vi "Lancing 2 Integ.vi"(0 "Image Out":T8(plugin-control), 1 "REF ROI":T4 {"Contours"."Type" items=["No Selection", "Point", "Line", "Rectangle", "Oval", "Polygon", "Free", "Annulus", "Unused2", "Unused3", "Broken Line", "Free Hand Line", "Rotated Rectangle"]}, 2 "Edge Options Ref ROI":T2={"Edge Polarity"=2, "Kernel Size"=5, "Width"=5, "Minimum Edge Strength"=50.0, "Interpolation Type"=enum."Bilinear Fixed", "Data Processing Method"=enum."Average"} {"Edge Polarity" items=["All Edges", "Rising Edges", "Falling Edges"]; "Minimum Edge Strength" format="%.2f"; "Width" step=2; "Kernel Size" step=2}, 3 "Search Direction Ref ROI":u32(ring)=2 items=["Left to Right", "Right to Left", "Top to Bottom", "Bottom to Top"], 4 "Line Options Ref ROI":T6={"Number of Lines"=1, "Type"=enum."First Edge Rake", "Min. Score"=10.0, "Max. Score"=1000.0, "Orientation"=0.0, "Angle Range"=30.0, "Angle Tolerance"=5.0, "Step Size"=3, "Min. SNR (db)"=0.0, "Min. Points (%)"=25.0, "Hough Iterations"=5} {"Min. Points (%)" min=0.0 max=100.0; "Min. SNR (db)" min=0.0; "Max. Score" min=0.0 max=1024.0; "Min. Score" min=0.0 max=1024.0 step=1.0}, 5 "Meas ROI 1":T4 {"Contours"."Type" items=["No Selection", "Point", "Line", "Rectangle", "Oval", "Polygon", "Free", "Annulus", "Unused2", "Unused3", "Broken Line", "Free Hand Line", "Rotated Rectangle"]}, 6 "Meas ROI 2":T4 {"Contours"."Type" items=["No Selection", "Point", "Line", "Rectangle", "Oval", "Polygon", "Free", "Annulus", "Unused2", "Unused3", "Broken Line", "Free Hand Line", "Rotated Rectangle"]}, 7 "error in (no error)":errorcluster, 8 "Calibrated Image":T8, 9 "Edge Options ROI 1":T2={"Edge Polarity"=2, "Kernel Size"=5, "Width"=5, "Minimum Edge Strength"=100.0, "Interpolation Type"=enum."Bilinear Fixed", "Data Processing Method"=enum."Average"} {"Edge Polarity" items=["All Edges", "Rising Edges", "Falling Edges"]; "Minimum Edge Strength" format="%.2f"; "Width" step=2; "Kernel Size" step=2}, 10 "Step Size ROI 1":u32=5, 11 "Process ROI 1":T1(ring), 12 "Scan Direction ROI 1":u16(ring)=3 items=["Left To Right", "Right To Left", "Top To Bottom", "Bottom To Top"], 13 "Process ROI 2":T1(ring), 14 "Step Size ROI 2":u32=1, 15 "OverlayOptions":T5, 16 "Edge Options ROI 2":T2={"Edge Polarity"=2, "Kernel Size"=9, "Width"=9, "Minimum Edge Strength"=50.0, "Interpolation Type"=enum."Bilinear Fixed", "Data Processing Method"=enum."Average"} {"Edge Polarity" items=["All Edges", "Rising Edges", "Falling Edges"]; "Minimum Edge Strength" format="%.2f"; "Width" step=2; "Kernel Size" step=2}, 17 "Scan Direction ROI 2":u16(ring)=3 items=["Left To Right", "Right To Left", "Top To Bottom", "Bottom To Top"]) -> (20 "Lancing 2":sgl, 27 "error out":errorcluster)   [LabVIEW 2019, in "Algorithm.lvclass"]
uses:
  FrameworkOverrides/Algorithm.lvclass
  <vilib>/vision/NI_Vision_Development_Module.lvlib
  <vilib>/vision/Image Controls.llb/IMAQ Image.ctl
  <vilib>/vision/Measure.llb/Edge Polarity.ctl
  <vilib>/vision/Measure.llb/Edge Options.ctl
  <vilib>/vision/Measure.llb/Straight Edge Process.ctl
  <vilib>/vision/Measure.llb/Straight Edge Options.ctl
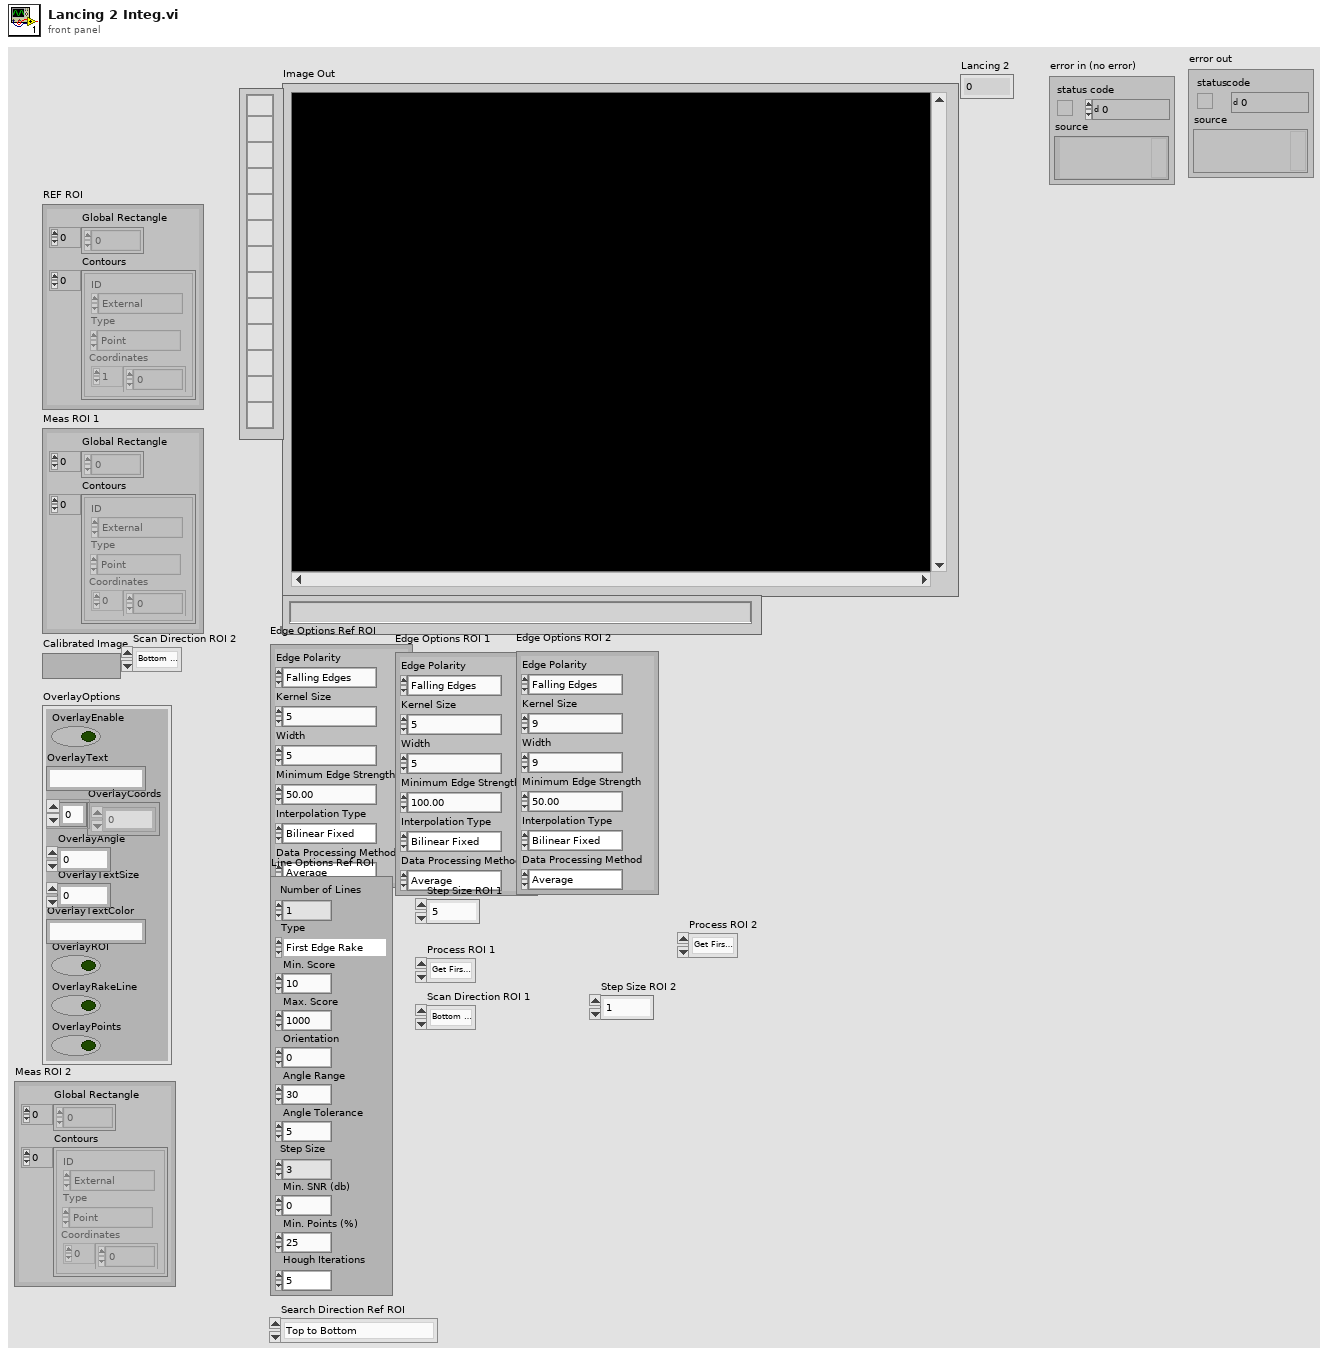
[diagram p1: front panel]
types:
  T1 = enum16{"Get First Edge", "Get First + Last Edge", "Get All Edges", "Get Best Edge"}
  T2 = typedef "Edge Options.ctl" = cluster{"Edge Polarity":T3, "Kernel Size":u32, "Width":u32, "Minimum Edge Strength":sgl, "Interpolation Type":enum32{"Zero Order", "Bilinear", "Quadratic", "Cubic", "Bilinear Fixed"}, "Data Processing Method":enum32{"Average", "Median"}}
  T3 = typedef "Edge Polarity.ctl" = u32
  T4 = cluster{"Global Rectangle":i32[], "Contours":cluster{"ID":enum32{"External", "Internal"}, "Type":u32, "Coordinates":i32[]}[]}
  T5 = cluster{"OverlayEnable":bool, "OverlayText":string, "OverlayCoords":i32[], "OverlayAngle":i32, "OverlayTextSize":i32, "OverlayTextColor":string, "OverlayROI":bool, "OverlayRakeLine":bool, "OverlayPoints":bool}
  T6 = typedef "Straight Edge Options.ctl" = cluster{"Number of Lines":i32, "Type":T7, "Min. Score":dbl, "Max. Score":dbl, "Orientation":dbl, "Angle Range":dbl, "Angle Tolerance":dbl, "Step Size":u32, "Min. SNR (db)":dbl, "Min. Points (%)":dbl, "Hough Iterations":i32}
  T7 = typedef "Straight Edge Process.ctl" = enum32{"First Edge Rake", "Best Edge Rake", "Hough Edge Rake", "First Edge Projection", "Best Edge Projection"}
  T8 = typedef "IMAQ Image.ctl" = refnum<image>
  T9 = cluster{"Point 1":cluster{"X":sgl, "Y":sgl}, "Point 2":cluster{"X":sgl, "Y":sgl}}
  T10 = typedef "IMAQ Rectangle" = cluster{"Left":i32, "Top":i32, "Right":i32, "Bottom":i32, "Rotation":dbl}
  T11 = cluster{"Point1 (Pixels)":cluster{"X":sgl, "Y":sgl}, "Point2 (Pixels)":cluster{"X":sgl, "Y":sgl}, "Point1 (Real-World)":cluster{"X":sgl, "Y":sgl}, "Point2 (Real-World)":cluster{"X":sgl, "Y":sgl}, "Angle (Pixel)":dbl, "Angle (Real-World)":dbl, "Score":dbl, "Straightness":dbl, "Average SNR (db)":dbl, "Calibration Valid":bool}[]
  T12 = typedef "Search Line.ctl" = cluster{"Start Point":cluster{"X":sgl, "Y":sgl}, "End Point":cluster{"X":sgl, "Y":sgl}, "Edge Info":T13[], "Edge Map":dbl[], "Calibration Valid":bool}
  T13 = typedef "Edge New.ctl" = cluster{"Location (Pixel)":cluster{"X":sgl, "Y":sgl}, "Location (Real-World)":cluster{"X":sgl, "Y":sgl}, "Distance (Pixel)":dbl, "Distance (Real-World)":dbl, "Strength":dbl, "Noise":dbl, "Rising?":bool}
  T14 = cluster{"Point1 (Pixels)":cluster{"X":sgl, "Y":sgl}, "Point2 (Pixels)":cluster{"X":sgl, "Y":sgl}, "Point1 (Real-World)":cluster{"X":sgl, "Y":sgl}, "Point2 (Real-World)":cluster{"X":sgl, "Y":sgl}, "Angle (Pixel)":dbl, "Angle (Real-World)":dbl, "Score":dbl, "Straightness":dbl, "Average SNR (db)":dbl, "Calibration Valid":bool}
  T15 = typedef "ROI Descriptor" = cluster{"Global Rectangle":i32[], "Contours":cluster{"ID":enum32{"External", "Internal"}, "Type":u32, "Coordinates":i32[]}[]}
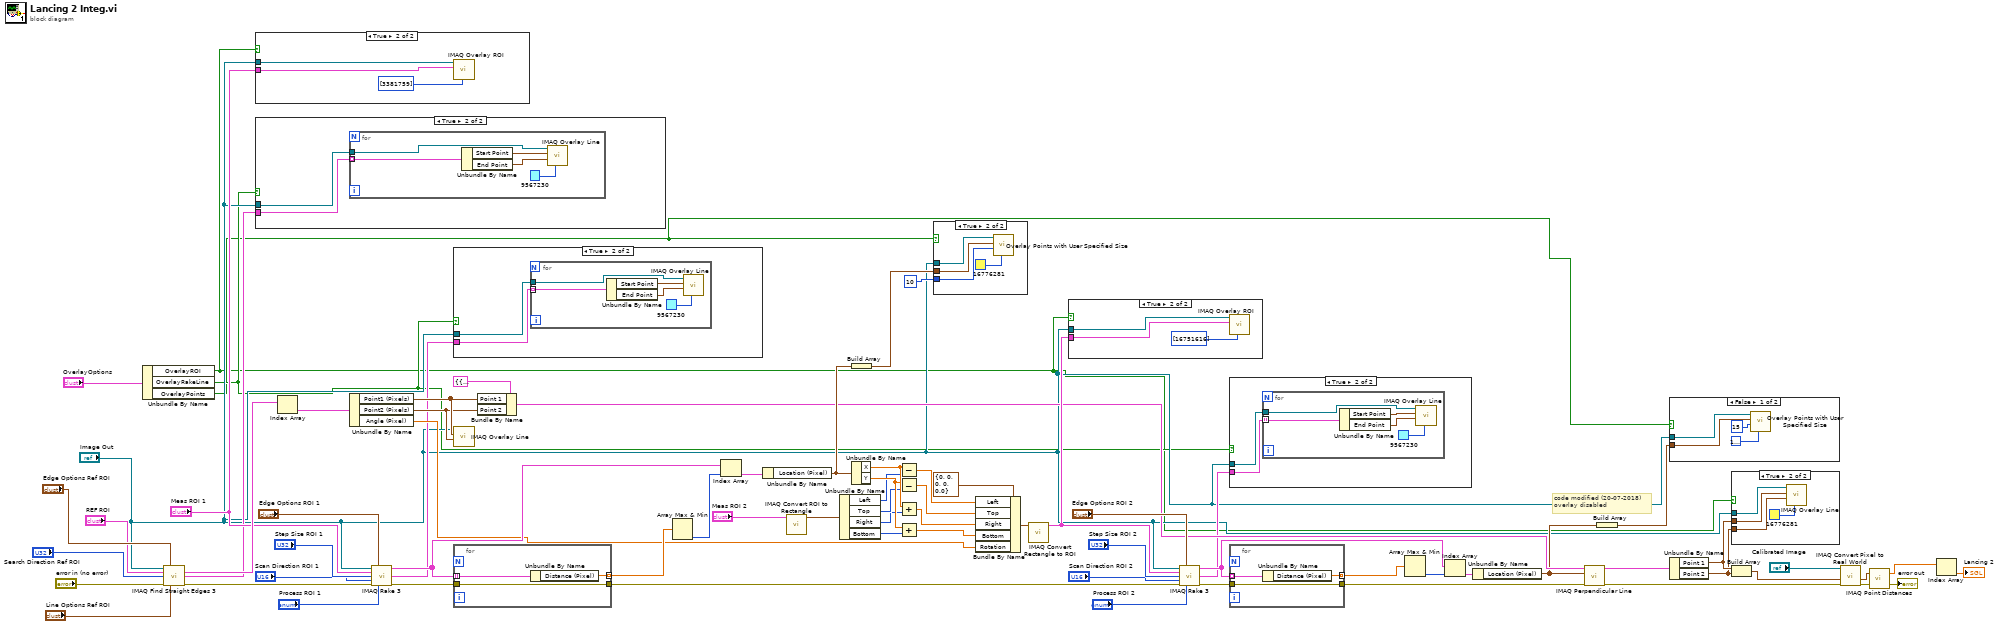
[diagram p0: block diagram]
diagram:
  # "code modified (20-07-2018)\noverlay disabled"
  n1 = Unbundle By Name("OverlayOptions") -> ("OverlayROI"=w2:bool, "OverlayRakeLine"=w4:bool, "OverlayPoints"=w3:bool)
  n2 = call "IMAQ Find Straight Edges 3"("Image"="Image Out", "Edge Options"="Edge Options Ref ROI", "ROI Descriptor"="REF ROI", "Search Direction"="Search Direction Ref ROI", "error in (no error)"="error in (no error)", "Line Options"="Line Options Ref ROI") -> ("Straight Edges"=w71:T11, "Search Lines Information"=w7:T12[], "error out"=w66:errorcluster)  [unwired: 5 in, 2 out]
  n3 = case shown="True" w2 {
    tunnel: "Meas ROI 1" -> [_ w76]
    tunnel: "Image Out" -> [_ w75]
    frame False {
    }
    frame True {
      n4 = call "IMAQ Overlay ROI"("Colors (Green)"=u32[] [3381759], "ROI Descriptor"=w76, "Image"=w75) -> ()  [unwired: 7 in, 2 out]
    }
  }
  n5 = case shown="True" w4 {
    tunnel: "Image Out" -> [_ w78]
    tunnel: w7 -> [_ w77]
    frame False {
    }
    frame True {
      n6 = for {
        tunnel: w77 -> [w83] mode=indexing
        tunnel: w78 -> [w79]
        n7 = Unbundle By Name(w83) -> ("Start Point"=w82:cluster{"X":sgl, "Y":sgl}, "End Point"=w81:cluster{"X":sgl, "Y":sgl})
        n8 = call "IMAQ Overlay Line"("Color"=u32 9567230, "End Point"=w81, "Start Point"=w82, "Image"=w79) -> ()  [unwired: 6 in, 2 out]
      }
    }
  }
  n9 = Index Array(array=w71) -> (element=w70:T14)  [unwired: 1 in]
  n10 = Unbundle By Name(w70) -> ("Point1 (Pixels)"=w33:cluster{"X":sgl, "Y":sgl}, "Point2 (Pixels)"=w32:cluster{"X":sgl, "Y":sgl}, "Angle (Pixel)"=w54:dbl)
  n11 = call "IMAQ Rake 3"("Image"="Image Out", "Edge Options"="Edge Options ROI 1", "ROI Descriptor"="Meas ROI 1", "Step Size"="Step Size ROI 1", "Scan Direction"="Scan Direction ROI 1", "error in (no error)"=w66, "Process"="Process ROI 1") -> ("First Edges"=w62:T13[], "Search Lines"=w8:T12[], "error out"=w57:errorcluster)  [unwired: 5 in, 1 out]
  n12 = case shown="True" w4 {
    tunnel: w8 -> [_ w85]
    tunnel: "Image Out" -> [_ w84]
    frame False {
    }
    frame True {
      n13 = for {
        tunnel: w85 -> [w90] mode=indexing
        tunnel: w84 -> [w86]
        n14 = Unbundle By Name(w90) -> ("Start Point"=w89:cluster{"X":sgl, "Y":sgl}, "End Point"=w88:cluster{"X":sgl, "Y":sgl})
        n15 = call "IMAQ Overlay Line"("Color"=u32 9567230, "End Point"=w88, "Start Point"=w89, "Image"=w86) -> ()  [unwired: 6 in, 2 out]
      }
    }
  }
  n16 = call "IMAQ Overlay Line"("End Point"=w32, "Start Point"=w33, "Image"="Image Out") -> ()  [unwired: 7 in, 2 out]
  n17 = for {
    tunnel: w62 -> [w93] mode=indexing
    tunnel: [w92] -> w63 mode=indexing
    tunnel: w57 -> [w91]
    tunnel: [w91] -> w42
    n18 = Unbundle By Name(w93) -> ("Distance (Pixel)"=w92:dbl)
  }
  n19 = Bundle By Name(cluster=T9 {"Point 1"={"X"=0.0, "Y"=0.0}, "Point 2"={"X"=0.0, "Y"=0.0}} ("Line"), "Point 1"=w33, "Point 2"=w32) -> (w34:T9)
  n20 = Array Max & Min(array=w63) -> (min index (indices)=w61:i32)  [unwired: 3 out]
  n21 = Index Array(array=w62, index=w61) -> (element=w60:T13)
  n22 = Unbundle By Name(w60) -> ("Location (Pixel)"=w53:cluster{"X":sgl, "Y":sgl})
  n23 = call "IMAQ Convert ROI to Rectangle"("ROI Descriptor"="Meas ROI 2") -> ("Rectangle"=w14:T10)  [unwired: 8 in, 1 out]
  n24 = Unbundle By Name(w14) -> ("Left"=w13:i32, "Top"=w12:i32, "Right"=w11:i32, "Bottom"=w10:i32)
  n25 = Build Array(w53) -> (w59:cluster{"X":sgl, "Y":sgl}[])
  n26 = Unbundle By Name(w53) -> ("X"=w39:sgl, "Y"=w37:sgl)
  n27 = Subtract(x=w39, y=w13) -> (x-y=w55:sgl)
  n28 = Subtract(x=w37, y=w12) -> (x-y=w40:sgl)
  n29 = Add(x=w39, y=w11) -> (x+y=w38:sgl)
  n30 = Add(x=w37, y=w10) -> (x+y=w36:sgl)
  n31 = case shown="True" w3 {
    tunnel: w59 -> [_ w97]
    tunnel: u32 10 ("Point Diameter (5)") -> [_ w95]
    tunnel: "Image Out" -> [_ w94]
    frame False {
    }
    frame True {
      n32 = call "Overlay Points with User Specified Size.vi"("Color"=u32 16776281, "Point Diameter (5)"=w95, "Points"=w97, "Image In"=w94) -> ()  [unwired: 6 in, 2 out]
    }
  }
  n33 = Bundle By Name(cluster=T10 {"Left"=0, "Top"=0, "Right"=0, "Bottom"=0, "Rotation"=0.0} ("Rectangle"), "Left"=w55, "Top"=w40, "Right"=w38, "Bottom"=w36, "Rotation"=w54) -> (w52:T10)
  n34 = call "IMAQ Convert Rectangle to ROI"("Rectangle"=w52) -> ("ROI Descriptor"=w41:T15)  [unwired: 8 in, 1 out]
  n35 = case shown="True" w2 {
    tunnel: w41 -> [_ w100]
    tunnel: "Image Out" -> [_ w98]
    frame False {
    }
    frame True {
      n36 = call "IMAQ Overlay ROI"("Colors (Green)"=u32[] [16751616], "ROI Descriptor"=w100, "Image"=w98) -> ()  [unwired: 7 in, 2 out]
    }
  }
  n37 = call "IMAQ Rake 3"("Image"="Image Out", "Edge Options"="Edge Options ROI 2", "ROI Descriptor"=w41, "Step Size"="Step Size ROI 2", "Scan Direction"="Scan Direction ROI 2", "error in (no error)"=w42, "Process"="Process ROI 2") -> ("First Edges"=w47:T13[], "Search Lines"=w6:T12[], "error out"=w51:errorcluster)  [unwired: 5 in, 1 out]
  n38 = case shown="True" w4 {
    tunnel: "Image Out" -> [_ w102]
    tunnel: w6 -> [_ w101]
    frame False {
    }
    frame True {
      n39 = for {
        tunnel: w101 -> [w107] mode=indexing
        tunnel: w102 -> [w103]
        n40 = Unbundle By Name(w107) -> ("Start Point"=w106:cluster{"X":sgl, "Y":sgl}, "End Point"=w105:cluster{"X":sgl, "Y":sgl})
        n41 = call "IMAQ Overlay Line"("Color"=u32 9567230, "End Point"=w105, "Start Point"=w106, "Image"=w103) -> ()  [unwired: 6 in, 2 out]
      }
    }
  }
  n42 = for {
    tunnel: w47 -> [w110] mode=indexing
    tunnel: [w109] -> w46 mode=indexing
    tunnel: w51 -> [w108]
    tunnel: [w108] -> w29
    n43 = Unbundle By Name(w110) -> ("Distance (Pixel)"=w109:dbl)
  }
  n44 = Array Max & Min(array=w46) -> (min index (indices)=w45:i32)  [unwired: 3 out]
  n45 = Index Array(array=w47, index=w45) -> (element=w44:T13)
  n46 = Unbundle By Name(w44) -> ("Location (Pixel)"=w31:cluster{"X":sgl, "Y":sgl})
  n47 = call "IMAQ Perpendicular Line"("error in (no error)"=w29, "Point"=w31, "Line"=w34) -> ("error out"=w22:errorcluster, "Perpendicular Line"=w30:T9)  [unwired: 6 in, 1 out]
  n48 = Build Array(w31) -> (w43:cluster{"X":sgl, "Y":sgl}[])
  n49 = case shown="False" w3 {
    tunnel: w43 -> [w114 _]
    tunnel: "Image Out" -> [w111 _]
    frame False {
      n50 = call "Overlay Points with User Specified Size.vi"("Color"=u32 16777226, "Point Diameter (5)"=u32 15, "Points"=w114, "Image In"=w111) -> ()  [unwired: 6 in, 2 out]
    }
    frame True {
    }
  }
  n51 = Unbundle By Name(w30) -> ("Point 1"=w25:cluster{"X":sgl, "Y":sgl}, "Point 2"=w24:cluster{"X":sgl, "Y":sgl})
  n52 = case shown="True" w2 {
    tunnel: w25 -> [_ w117]
    tunnel: w24 -> [_ w116]
    tunnel: "Image Out" -> [_ w115]
    frame False {
    }
    frame True {
      n53 = call "IMAQ Overlay Line"("Color"=u32 16776281, "End Point"=w116, "Start Point"=w117, "Image"=w115) -> ()  [unwired: 6 in, 2 out]
    }
  }
  n54 = Build Array(w25, w24) -> (w23:cluster{"X":sgl, "Y":sgl}[])
  n55 = call "IMAQ Convert Pixel to Real World"("error in (no error)"=w22, "Array of Pixel Coordinates"=w23, "Calibrated Image"="Calibrated Image") -> ("error out"=w18:errorcluster, "Array of Real World Coordinates"=w21:cluster{"X":sgl, "Y":sgl}[])  [unwired: 3 in, 4 out]
  n56 = call "IMAQ Point Distances"("Points"=w21, "error in (no error)"=w18) -> ("Distances"=w20:sgl[], "error out"=→"error out":errorcluster)  [unwired: 3 in]
  n57 = Index Array(array=w20) -> (element=→"Lancing 2":sgl)  [unwired: 1 in]
